vi "Apply Config.vi"(8 "error in (no error)":errorcluster, 10 "Config":T1={"Process Model"={"Seq Path"=""}, "Break On First Step?"=FALSE, "Break On Step Failure?"=TRUE, "Break On Sequence Failure?"=FALSE, "Tracing Enabled?"=TRUE, "Goto Cleanup on Sequence Failure?"=TRUE}, 11 "teststand-api in":refnum<class "teststand-api.lvclass">) -> (0 "error out":errorcluster, 3 "teststand-api out":refnum<class "teststand-api.lvclass">)   [LabVIEW 2014, in "teststand-api.lvlib" / "teststand-api.lvclass"]
uses:
  teststand-api.lvclass
  Config Argument--cluster.ctl
  Process Model--cluster.ctl
  teststand-api.lvclass/teststand-api.ctl
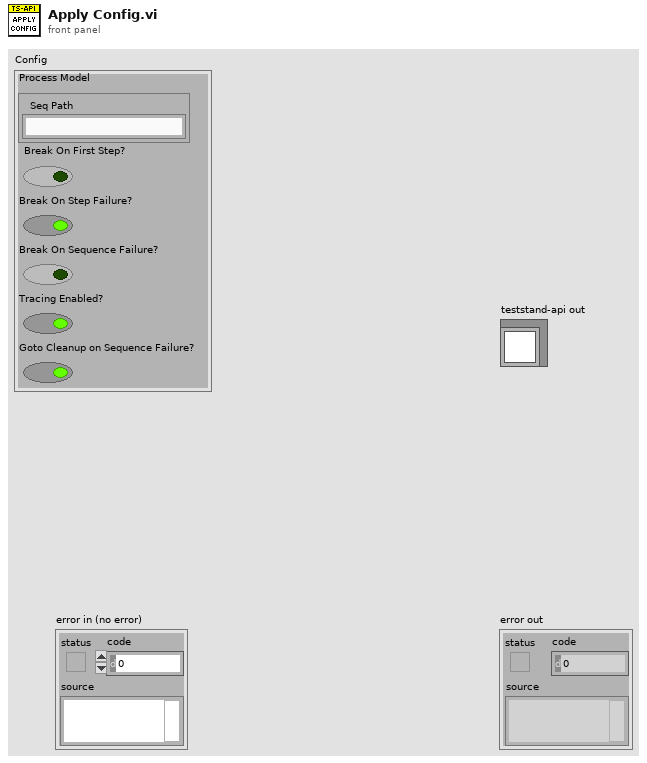
[diagram p1: front panel]
types:
  T1 = typedef "teststand-api.lvlib/teststand-api.lvclass/Config Argument--cluster.ctl" = cluster{"Process Model":T2, "Break On First Step?":bool, "Break On Step Failure?":bool, "Break On Sequence Failure?":bool, "Tracing Enabled?":bool, "Goto Cleanup on Sequence Failure?":bool}
  T2 = typedef "teststand-api.lvlib/teststand-api.lvclass/Process Model--cluster.ctl" = cluster{"Seq Path":string}
  T3 = typedef "teststand-api.lvlib/teststand-api.lvclass/Manager Controls Argument--cluster.ctl" = cluster{"App Manager":refnum<k7>, "Seq Manager":refnum<k7>, "Exec Manager":refnum<k7>}
  T4 = typedef "teststand-api.lvlib/teststand-api.lvclass/Other Refs Argument--cluster.ctl" = cluster{"TS Engine":refnum<k7>, "Top Level VI ":refnum<vi>, "Sequence File":refnum<k7>, "Execution":refnum<k7>, "Process Model Seq":refnum<k7>, "Process Model":T2}
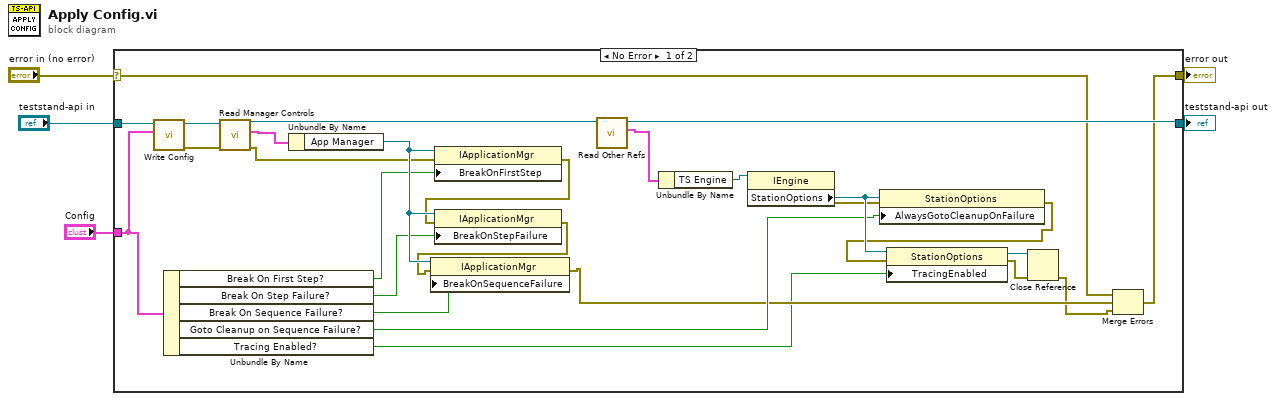
[diagram p0: block diagram]
diagram:
  n1 = case shown="No Error" "error in (no error)" {
    selector: "error in (no error)" -> [w9 w34]
    tunnel: [w7 w34] -> w4
    tunnel: [w23 w33] -> w2
    tunnel: "teststand-api in" -> [w32 w33]
    tunnel: "Config" -> [w28 _]
    frame No Error {
      n2 = call "Write Config.vi"("Config"=w28, "teststand-api in"=w32) -> ("error out"=w10:errorcluster, "teststand-api out"=w31:refnum<class "teststand-api.lvclass">)  [unwired: 8 in]
      n3 = Unbundle By Name(w28) -> ("Break On First Step?"=w27:bool, "Break On Step Failure?"=w26:bool, "Break On Sequence Failure?"=w25:bool, "Goto Cleanup on Sequence Failure?"=w18:bool, "Tracing Enabled?"=w6:bool)
      n4 = call-dynamic "Read Manager Controls.vi"("error in (no error)"=w10, "teststand-api in"=w31) -> ("error out"=w11:errorcluster, "Manager Controls"=w30:T3, "teststand-api out"=w24:refnum<class "teststand-api.lvclass">)  [unwired: 7 in]
      n5 = Unbundle By Name(w30) -> ("App Manager"=w29:refnum<k7>)
      n6 = property class="IApplicationMgr"(reference=w29, error in=w11, "BreakOnFirstStep"=w27) -> (error out=w17:errorcluster)  [unwired: 1 out]
      n7 = property class="IApplicationMgr"(reference=w29, error in=w17, "BreakOnStepFailure"=w26) -> (error out=w16:errorcluster)  [unwired: 1 out]
      n8 = property class="IApplicationMgr"(reference=w29, error in=w16, "BreakOnSequenceFailure"=w25) -> (error out=w12:errorcluster)  [unwired: 1 out]
      n9 = call-dynamic "Read Other Refs.vi"("teststand-api in"=w24) -> ("Refs"=w22:T4, "teststand-api out"=w23:refnum<class "teststand-api.lvclass">)  [unwired: 8 in, 1 out]
      n10 = Unbundle By Name(w22) -> ("TS Engine"=w21:refnum<k7>)
      n11 = property class="IEngine"(reference=w21) -> (error out=w19:errorcluster, "StationOptions"=w20:refnum<k7>)  [unwired: 1 in, 1 out]
      n12 = property class="StationOptions"(reference=w20, error in=w19, "AlwaysGotoCleanupOnFailure"=w18) -> (error out=w15:errorcluster)  [unwired: 1 out]
      n13 = property class="StationOptions"(reference=w20, error in=w15, "TracingEnabled"=w6) -> (reference out=w14:refnum<k7>, error out=w13:errorcluster)
      n14 = Close Reference(reference=w14, error in (no error)=w13) -> (error out=w8:errorcluster)
      n15 = Merge Errors(w9, w12, w8) -> (w7:errorcluster)
    }
    frame Error {
    }
  }
  "error out" <- w4
  "teststand-api out" <- w2
